vi "7.1 Button Latch.vi"(1 "Input":bool) -> (0 "Boolean":bool)   [LabVIEW 2011]
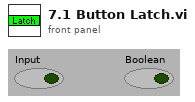
[diagram p1: front panel]
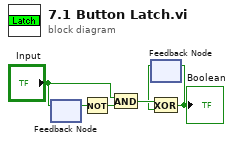
[diagram p0: block diagram]
diagram:
  n1 = feedback #1() -> (w1:bool)  [unwired: 1 in]
  n2 = feedback-in #1("Input") -> ()
  n3 = Not(x=w1) -> (.not. x?=w3:bool)
  n4 = And(x="Input", y=w3) -> (x .and. y?=w5:bool)
  n5 = feedback #2() -> (w4:bool)  [unwired: 1 in]
  n6 = Exclusive Or(1:w4, 2:w5) -> (0:w6:bool)
  "Boolean" <- w6
  n7 = feedback-in #2(w6) -> ()
